vi "Grafici MANAGER.vi"() -> ()   [LabVIEW 2019]
uses:
  TypeDef/Definizione_Grafico_REPORT.ctl
  TypeDef/Definizione_plot.ctl
  Global percorso impostazioni.vi
panel:
  in  "proponi plot":bool
  in  "SALVA plots":bool
  in  "SALVA GRAFICI":bool
  in  "exit":bool
  out "deleted portion":T1[](array[typedef]) {"PLOT"."GRANDEZZA Y" items=["Banco", "Anno", "Numero", "N° tabella", "Misura", "Tipo prova", "Progressivo Acq", "tempo[h:m:s]", "tempo acq[min]", "f [Hz]", "Uav [V]", "Iav [A]", "Tq [Nm]", "n [rpm]", "P1 [kW]", "P1 n[kW]", "Q [m3/h]", "Q n[m3/h]", "Q [l/min]", "Q n[l/min]", "H1 [m]", "Dislivello [m]", "Hdinamica [m]", "HvAsp [m]", "HvMand [m]", "HvTot [m]", "H2 [m]", "Htot [m]", "Htot n[m]", "P3 (Phyd) [kW]", "P3 (Phyd) n[kW]", "P2 [kW]", "P2 n[kW]", "P2 n ps[kW]", "eta motore [%]", "eta pompa [%]", "eta pompa n[%]", "eta gruppo [%]", "eta gruppo n[%]", "T acqua [°C]", "Densità liquido [kg/m3]", "P barometrica [mbar]", "pf", "Uch1 [V]", "Uch2 [V]", "Uch3 [V]", "Ich1 [A]", "Ich2 [A]", "Ich3 [A]", "Temp.amb[°C]", "Ru-w [ohm]", "DTavvolg. [°C]", "Tamb Freddo [°C]", "Ru-w Freddo [ohm]", "Tc1[°C]", "Tc2[°C]", "Tc3[°C]", "Tc4[°C]", "Tc5", "Tc6", "Tc7", "Tc8", "H1[Bar]", "H2[bar]", "P premist.[Bar]", "Pserb[bar]", "n°NPSH", "NPSH", "Htot Ref[m]", "NPSH_%caduta", "%caduta", "Qref [m3/h]", "MEI"]; "PLOT"."GRANDEZZA X" items=["Banco", "Anno", "Numero", "N° tabella", "Misura", "Tipo prova", "Progressivo Acq", "tempo[h:m:s]", "tempo acq[min]", "f [Hz]", "Uav [V]", "Iav [A]", "Tq [Nm]", "n [rpm]", "P1 [kW]", "P1 n[kW]", "Q [m3/h]", "Q n[m3/h]", "Q [l/min]", "Q n[l/min]", "H1 [m]", "Dislivello [m]", "Hdinamica [m]", "HvAsp [m]", "HvMand [m]", "HvTot [m]", "H2 [m]", "Htot [m]", "Htot n[m]", "P3 (Phyd) [kW]", "P3 (Phyd) n[kW]", "P2 [kW]", "P2 n[kW]", "P2 n ps[kW]", "eta motore [%]", "eta pompa [%]", "eta pompa n[%]", "eta gruppo [%]", "eta gruppo n[%]", "T acqua [°C]", "Densità liquido [kg/m3]", "P barometrica [mbar]", "pf", "Uch1 [V]", "Uch2 [V]", "Uch3 [V]", "Ich1 [A]", "Ich2 [A]", "Ich3 [A]", "Temp.amb[°C]", "Ru-w [ohm]", "DTavvolg. [°C]", "Tamb Freddo [°C]", "Ru-w Freddo [ohm]", "Tc1[°C]", "Tc2[°C]", "Tc3[°C]", "Tc4[°C]", "Tc5", "Tc6", "Tc7", "Tc8", "H1[Bar]", "H2[bar]", "P premist.[Bar]", "Pserb[bar]", "n°NPSH", "NPSH", "Htot Ref[m]", "NPSH_%caduta", "%caduta", "Qref [m3/h]", "MEI"]; "Assi grafico"."ASSE X" items=["X 1", "X 2"]; "Assi grafico"."ASSE Y" items=["Y 1", "Y 2", "Y 3", "Y 4"]}
  out "Array plot":T1[](array[typedef]) {"PLOT"."GRANDEZZA Y" items=["Banco", "Anno", "Numero", "N° tabella", "Misura", "Tipo prova", "Progressivo Acq", "tempo[h:m:s]", "tempo acq[min]", "f [Hz]", "Uav [V]", "Iav [A]", "Tq [Nm]", "n [rpm]", "P1 [kW]", "P1 n[kW]", "Q [m3/h]", "Q n[m3/h]", "Q [l/min]", "Q n[l/min]", "H1 [m]", "Dislivello [m]", "Hdinamica [m]", "HvAsp [m]", "HvMand [m]", "HvTot [m]", "H2 [m]", "Htot [m]", "Htot n[m]", "P3 (Phyd) [kW]", "P3 (Phyd) n[kW]", "P2 [kW]", "P2 n[kW]", "P2 n ps[kW]", "eta motore [%]", "eta pompa [%]", "eta pompa n[%]", "eta gruppo [%]", "eta gruppo n[%]", "T acqua [°C]", "Densità liquido [kg/m3]", "P barometrica [mbar]", "pf", "Uch1 [V]", "Uch2 [V]", "Uch3 [V]", "Ich1 [A]", "Ich2 [A]", "Ich3 [A]", "Temp.amb[°C]", "Ru-w [ohm]", "DTavvolg. [°C]", "Tamb Freddo [°C]", "Ru-w Freddo [ohm]", "Tc1[°C]", "Tc2[°C]", "Tc3[°C]", "Tc4[°C]", "Tc5", "Tc6", "Tc7", "Tc8", "H1[Bar]", "H2[bar]", "P premist.[Bar]", "Pserb[bar]", "n°NPSH", "NPSH", "Htot Ref[m]", "NPSH_%caduta", "%caduta", "Qref [m3/h]", "MEI"]; "PLOT"."GRANDEZZA X" items=["Banco", "Anno", "Numero", "N° tabella", "Misura", "Tipo prova", "Progressivo Acq", "tempo[h:m:s]", "tempo acq[min]", "f [Hz]", "Uav [V]", "Iav [A]", "Tq [Nm]", "n [rpm]", "P1 [kW]", "P1 n[kW]", "Q [m3/h]", "Q n[m3/h]", "Q [l/min]", "Q n[l/min]", "H1 [m]", "Dislivello [m]", "Hdinamica [m]", "HvAsp [m]", "HvMand [m]", "HvTot [m]", "H2 [m]", "Htot [m]", "Htot n[m]", "P3 (Phyd) [kW]", "P3 (Phyd) n[kW]", "P2 [kW]", "P2 n[kW]", "P2 n ps[kW]", "eta motore [%]", "eta pompa [%]", "eta pompa n[%]", "eta gruppo [%]", "eta gruppo n[%]", "T acqua [°C]", "Densità liquido [kg/m3]", "P barometrica [mbar]", "pf", "Uch1 [V]", "Uch2 [V]", "Uch3 [V]", "Ich1 [A]", "Ich2 [A]", "Ich3 [A]", "Temp.amb[°C]", "Ru-w [ohm]", "DTavvolg. [°C]", "Tamb Freddo [°C]", "Ru-w Freddo [ohm]", "Tc1[°C]", "Tc2[°C]", "Tc3[°C]", "Tc4[°C]", "Tc5", "Tc6", "Tc7", "Tc8", "H1[Bar]", "H2[bar]", "P premist.[Bar]", "Pserb[bar]", "n°NPSH", "NPSH", "Htot Ref[m]", "NPSH_%caduta", "%caduta", "Qref [m3/h]", "MEI"]; "Assi grafico"."ASSE X" items=["X 1", "X 2"]; "Assi grafico"."ASSE Y" items=["Y 1", "Y 2", "Y 3", "Y 4"]}
  out "Array grafici":T2[](array[typedef]) {"ASSE Y 5"."Decimali" min=0 max=6; "ASSE Y 4"."Decimali" min=0 max=6; "ASSE Y 3"."Decimali" min=0 max=6; "ASSE Y 2"."Decimali" min=0 max=6; "ASSE Y 1"."Decimali" min=0 max=6; "ASSE X 2"."Decimali" min=0 max=6; "ASSE X 1"."Decimali" min=0 max=6}
  in  "Tab Control":enum32{"GESTIONE GRAFICI"}(tab)
  in  "carica plot":bool
  in  "CARICA PLOT GRAFICI":bool
  in  "ELIMINA PLOT":bool
  in  "ELIMINA GRAFICO":bool
  in  "carica grafico":bool
  in  "lista grafici":i32(listbox) caption="LISTA GRAFICI ESISTENTI"
  in  "CREA GRAFICO":bool
  in  "GRAFICO":T2 {"ASSE Y 5"."Decimali" min=0 max=6; "ASSE Y 4"."Decimali" min=0 max=6; "ASSE Y 3"."Decimali" min=0 max=6; "ASSE Y 2"."Decimali" min=0 max=6; "ASSE Y 1"."Decimali" min=0 max=6; "ASSE X 2"."Decimali" min=0 max=6; "ASSE X 1"."Decimali" min=0 max=6}
  in  "PLOT":T1={"Assi grafico"={"ASSE Y"=0, "ASSE X"=0, "Colore x"=0, "Colore y"=0}, "TIPO COLLEGAMENTO"="", "PLOT"={"GRANDEZZA X"=0, "GRANDEZZA Y"=16, "COLORE PLOT"=0, "NOME PLOT"="", "Larghezza linea"=0, "stile linea"=0, "stile punto"=0}, "NOME GRAFICO"=""} {"PLOT"."GRANDEZZA Y" items=["Banco", "Anno", "Numero", "Ntabella", "Misura", "Tipo Prova", "ProgressivoAcq", "Descrizione", "Data_ora", "t. acq [h:m:s]", "t. acq [min]", "t. acq [s]", "n [rpm]", "f [Hz]", "U1[V]", "U2 [V]", "U3 [V]", "U123_media [V]", "I1[A]", "I2[A]", "I3[A]", "I123_media [A]*I", "I_123_sbil [%]", "pf", "P1 [W]", "P1 [kW]", "Q [VAR]", "Q [kVAR]", "S [VA]", "S [kVA]", "C [Nm]*C", "Cric [Nm]", "Cric\\Cnom", "Iric[A]", "Iric\\Inom", "P2_mecc [W]", "P2_mecc [kW]", "eta motore [%]", "Scorr[%]", "Tamb[°C]", "R1[ohm]", "R2[ohm]", "R3[ohm]", "DT_R1[°C]", "DT_R2[°C]", "DT_R3[°C]", "TambFreddo[°C]", "R1_freddo[ohm]", "R2_freddo[ohm]", "R3_freddo[ohm]", "DEO[mm\\s]", "DEO[ge]", "DEV[mm\\s]", "DEV[ge]", "NDEO[mm\\s]", "NDEO[ge]", "NDEV[mm\\s]", "NDEV[ge]", "ASS.[mm\\s]", "ASS.[ge]", "TC1[°C]", "TC2[°C]", "TC3[°C]"]; "PLOT"."GRANDEZZA X" items=["Banco", "Anno", "Numero", "Ntabella", "Misura", "Tipo Prova", "ProgressivoAcq", "Descrizione", "Data_ora", "t. acq [h:m:s]", "t. acq [min]", "t. acq [s]", "n [rpm]", "f [Hz]", "U1[V]", "U2 [V]", "U3 [V]", "U123_media [V]", "I1[A]", "I2[A]", "I3[A]", "I123_media [A]*I", "I_123_sbil [%]", "pf", "P1 [W]", "P1 [kW]", "Q [VAR]", "Q [kVAR]", "S [VA]", "S [kVA]", "C [Nm]*C", "Cric [Nm]", "Cric\\Cnom", "Iric[A]", "Iric\\Inom", "P2_mecc [W]", "P2_mecc [kW]", "eta motore [%]", "Scorr[%]", "Tamb[°C]", "R1[ohm]", "R2[ohm]", "R3[ohm]", "DT_R1[°C]", "DT_R2[°C]", "DT_R3[°C]", "TambFreddo[°C]", "R1_freddo[ohm]", "R2_freddo[ohm]", "R3_freddo[ohm]", "DEO[mm\\s]", "DEO[ge]", "DEV[mm\\s]", "DEV[ge]", "NDEO[mm\\s]", "NDEO[ge]", "NDEV[mm\\s]", "NDEV[ge]", "ASS.[mm\\s]", "ASS.[ge]", "TC1[°C]", "TC2[°C]", "TC3[°C]"]; "Assi grafico"."ASSE X" items=["RPM"]; "Assi grafico"."ASSE Y" items=["C[Nm]"]}
  in  "lista plot":i32(listbox) caption="LISTA PLOT"
  in  "Add plot":bool
  in  "Y Scale.Visible":bool
  in  "Active Y Scale":i32
  in  "X Scale.Visible":bool
  in  "Active X Scale":i32
  out "CURVE IDRAULICHE QH":cluster{"X":dbl[], "Y":dbl[]}[](graph)
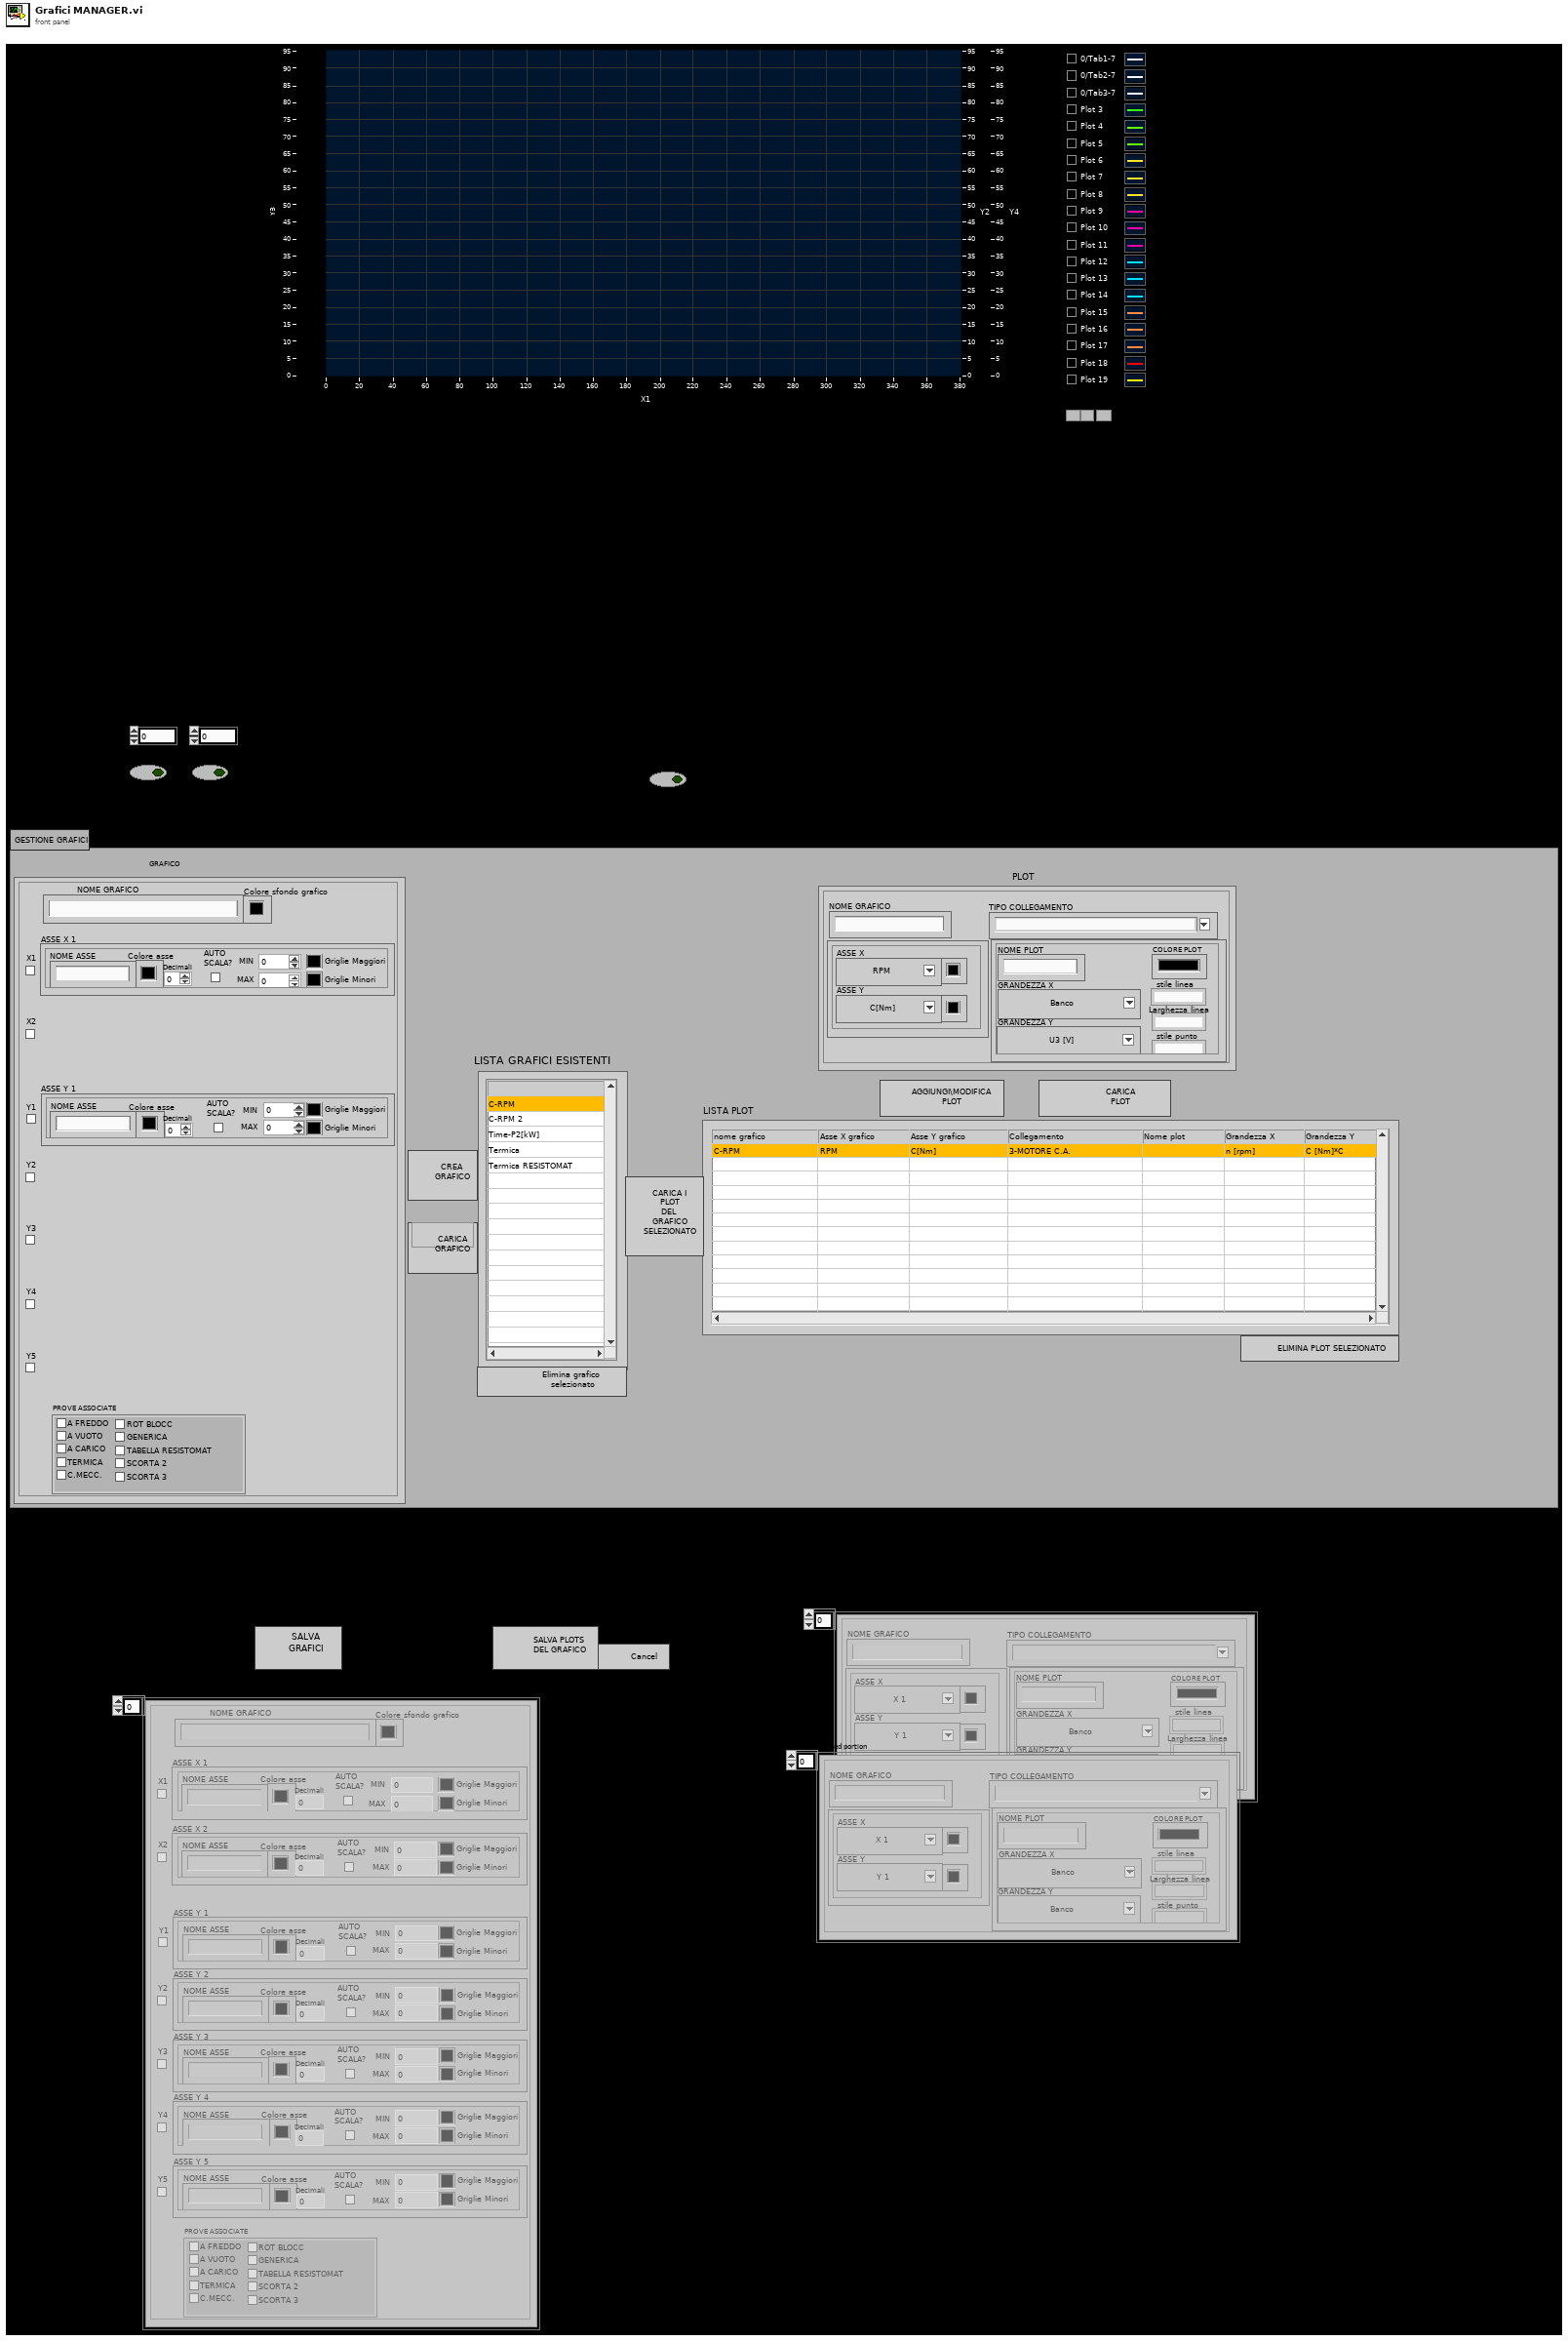
[diagram p1: front panel]
types:
  T1 = typedef "Definizione_plot.ctl" = cluster{"Assi grafico":cluster{"ASSE Y":u16, "ASSE X":u16, "Colore x":u32, "Colore y":u32}, "TIPO COLLEGAMENTO":string, "PLOT":cluster{"GRANDEZZA X":u16, "GRANDEZZA Y":u16, "COLORE PLOT":u32, "NOME PLOT":string, "Larghezza linea":u16, "stile linea":u16, "stile punto":u16}, "NOME GRAFICO":string}
  T2 = typedef "Definizione_Grafico_REPORT.ctl" = cluster{"ASSE X 1":cluster{"NOME ASSE":string, "AUTO\nSCALA?":bool, "MIN":dbl, "MAX":dbl, "Colore asse":u32, "Griglie Maggiori":u32, "Griglie Minori":u32, "Decimali":i8}, "ASSE X 2":cluster{"NOME ASSE":string, "AUTO\nSCALA?":bool, "MIN":dbl, "MAX":dbl, "Colore asse":u32, "Griglie Maggiori":u32, "Griglie Minori":u32, "Decimali":i8}, "ASSE Y 1":cluster{"NOME ASSE":string, "AUTO\nSCALA?":bool, "MIN":dbl, "MAX":dbl, "Colore asse":u32, "Griglie Maggiori":u32, "Griglie Minori":u32, "Decimali":i8}, "ASSE Y 2":cluster{"NOME ASSE":string, "AUTO\nSCALA?":bool, "MIN":dbl, "MAX":dbl, "Colore asse":u32, "Griglie Maggiori":u32, "Griglie Minori":u32, "Decimali":i8}, "ASSE Y 3":cluster{"NOME ASSE":string, "AUTO\nSCALA?":bool, "MIN":dbl, "MAX":dbl, "Colore asse":u32, "Griglie Maggiori":u32, "Griglie Minori":u32, "Decimali":i8}, "ASSE Y 4":cluster{"NOME ASSE":string, "AUTO\nSCALA?":bool, "MIN":dbl, "MAX":dbl, "Colore asse":u32, "Griglie Maggiori":u32, "Griglie Minori":u32, "Decimali":i8}, "X1":bool, "X2":bool, "Y1":bool, "Y2":bool, "Y3":bool, "Y4":bool, "NOME GRAFICO":string, "PROVE ASSOCIATE":cluster{"A FREDDO":bool, "A VUOTO":bool, "A CARICO":bool, "TERMICA":bool, "C.MECC.":bool, "ROT BLOCC":bool, "GENERICA":bool, "TABELLA RESISTOMAT":bool, "SCORTA 2":bool, "SCORTA 3":bool}, "ASSE Y 5":cluster{"NOME ASSE":string, "AUTO\nSCALA?":bool, "MIN":dbl, "MAX":dbl, "Colore asse":u32, "Griglie Maggiori":u32, "Griglie Minori":u32, "Decimali":i8}, "Y5":bool, "Colore sfondo grafico":u32}
  T3 = enum16{"open", "replace", "create", "open or create", "replace or create", "replace or create with confirmation"}
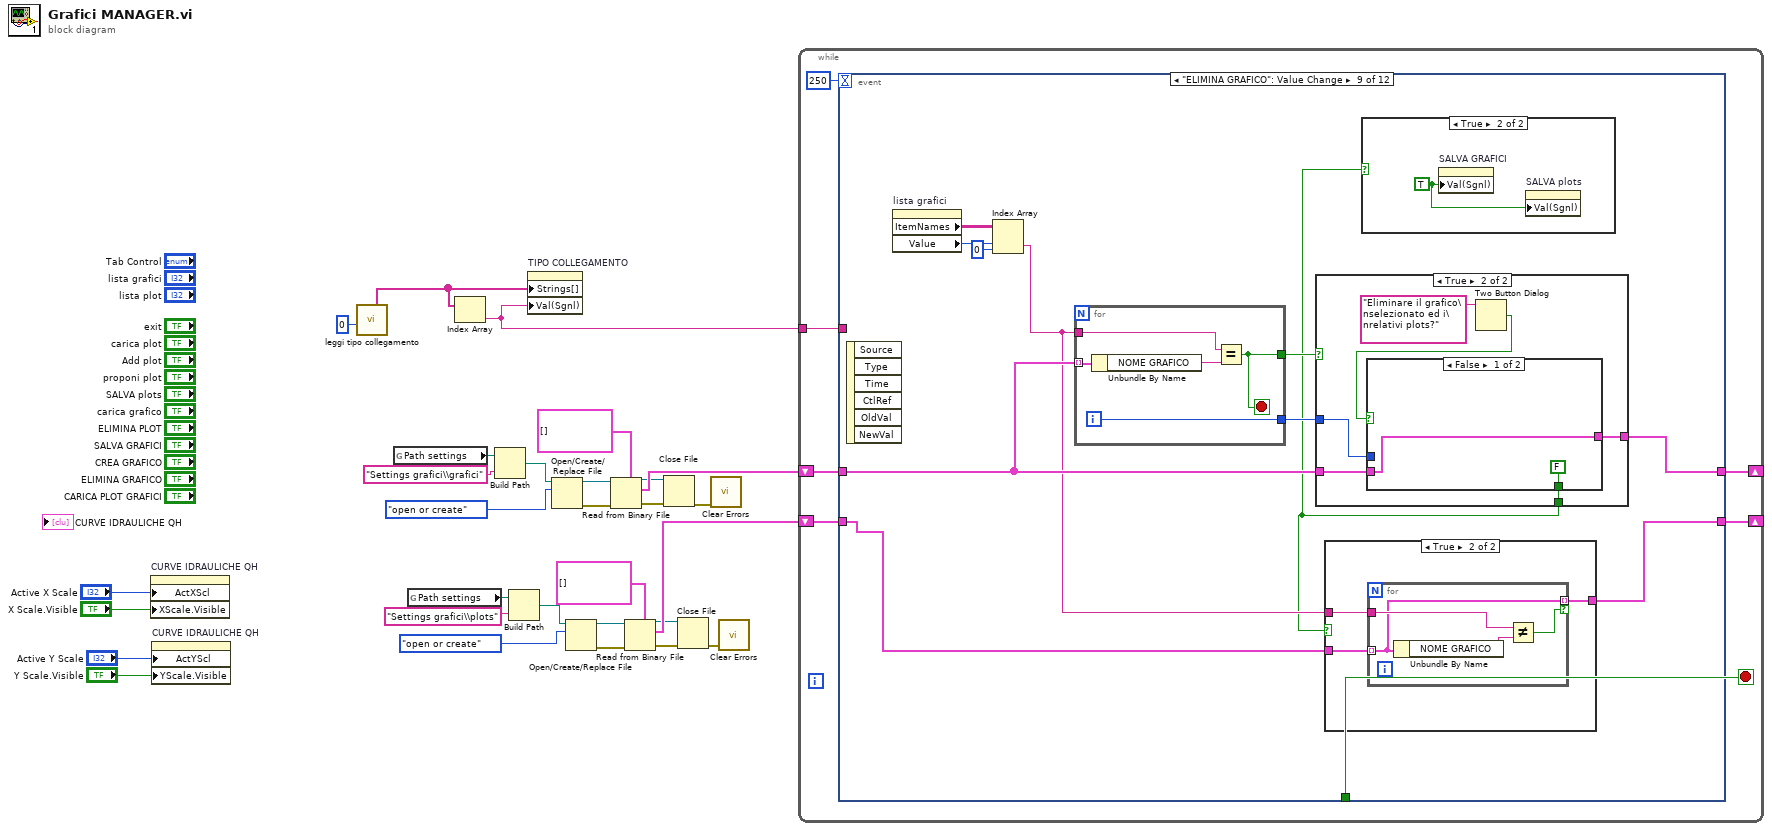
[diagram p0: block diagram]
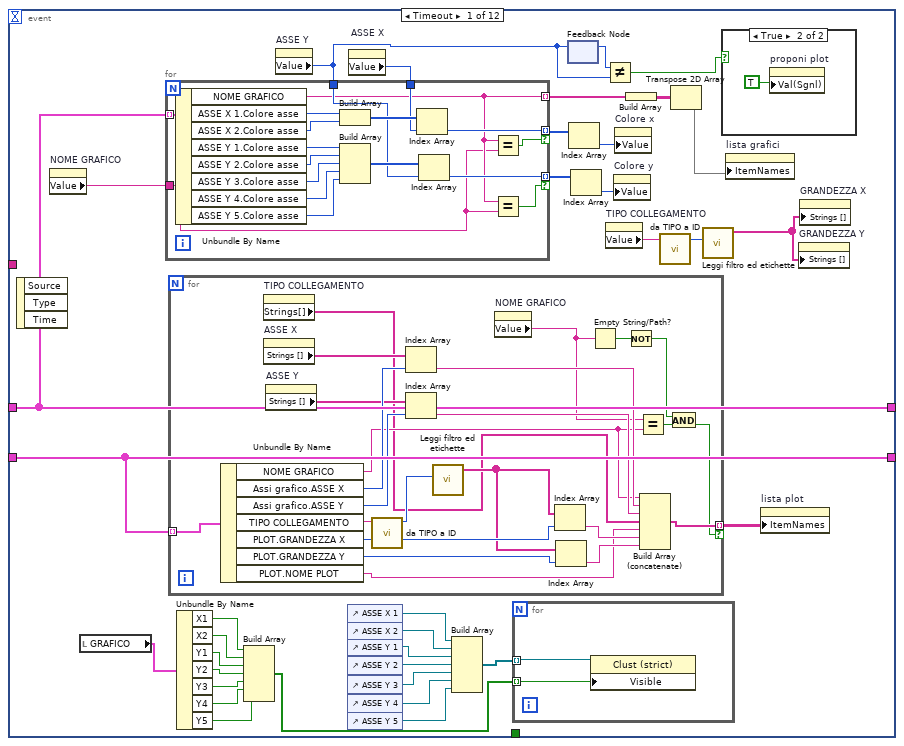
[diagram p2: hidden frame]
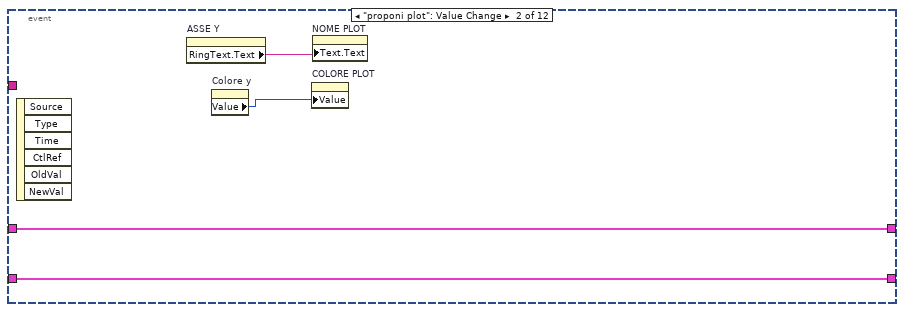
[diagram p4: hidden frame]
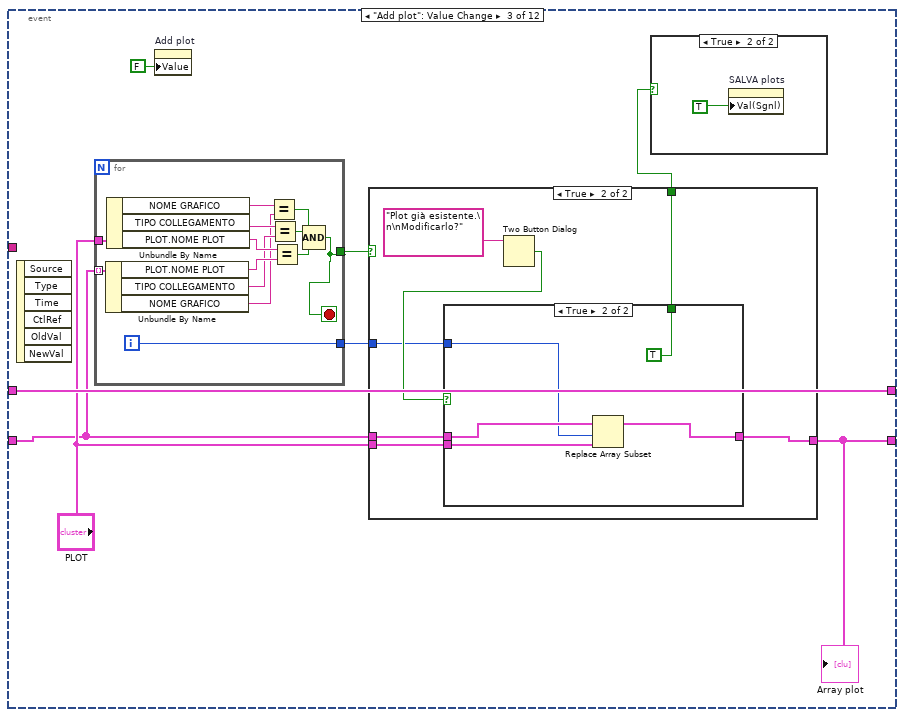
[diagram p5: hidden frame]
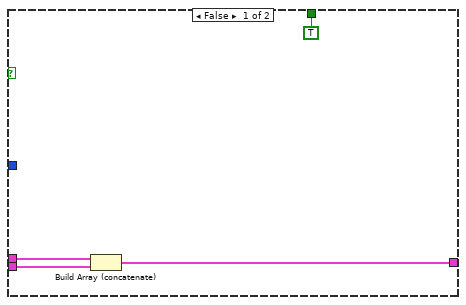
[diagram p7: hidden frame]
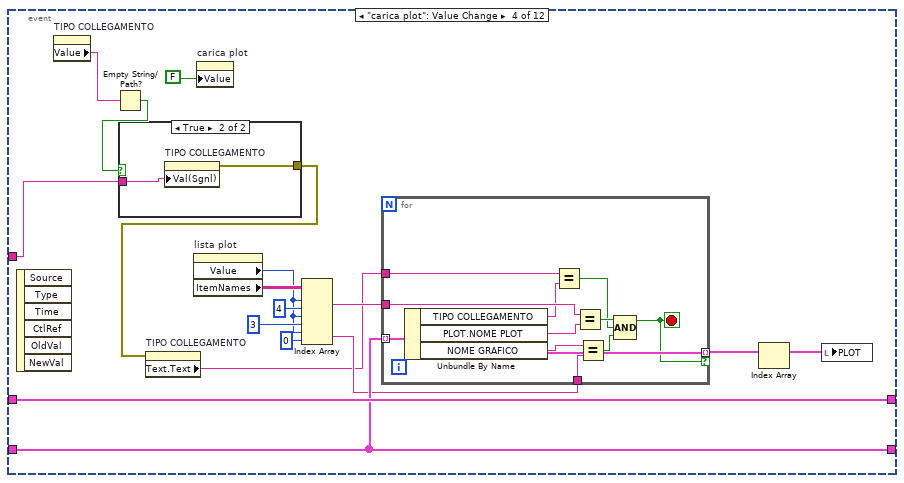
[diagram p9: hidden frame]
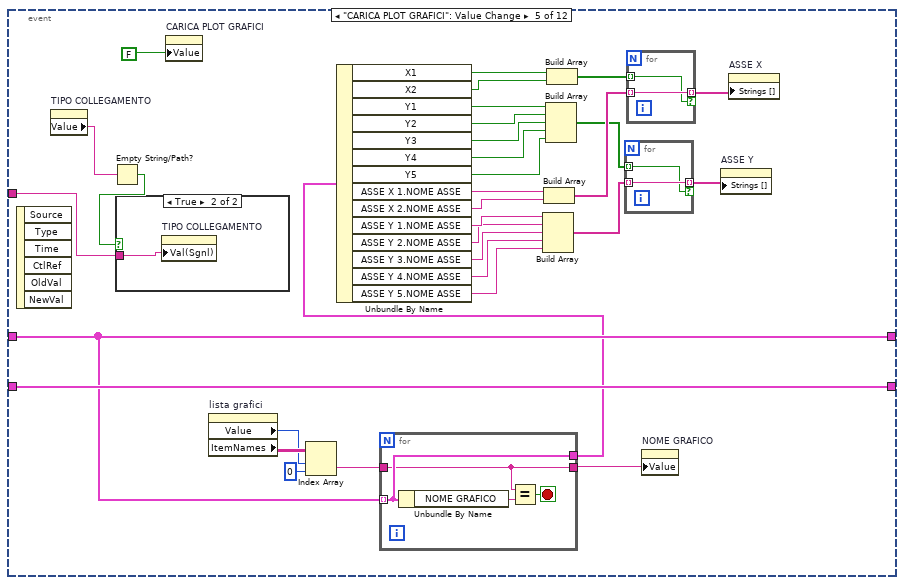
[diagram p11: hidden frame]
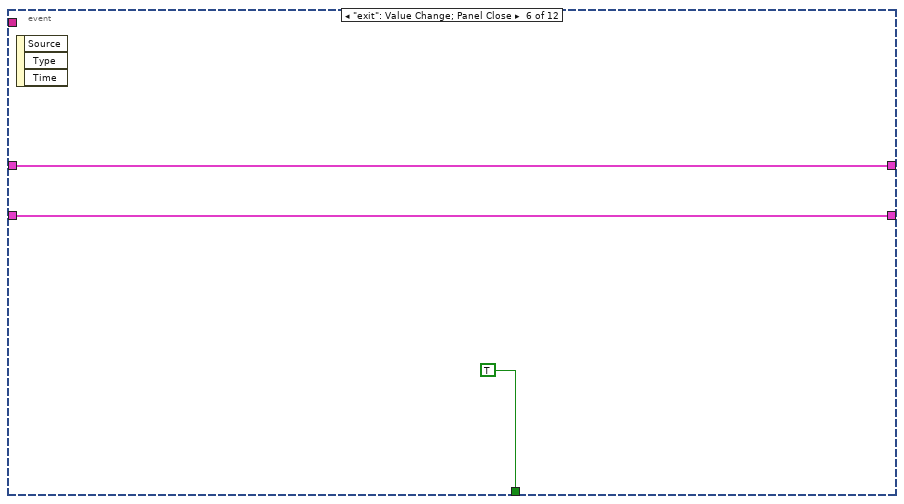
[diagram p13: hidden frame]
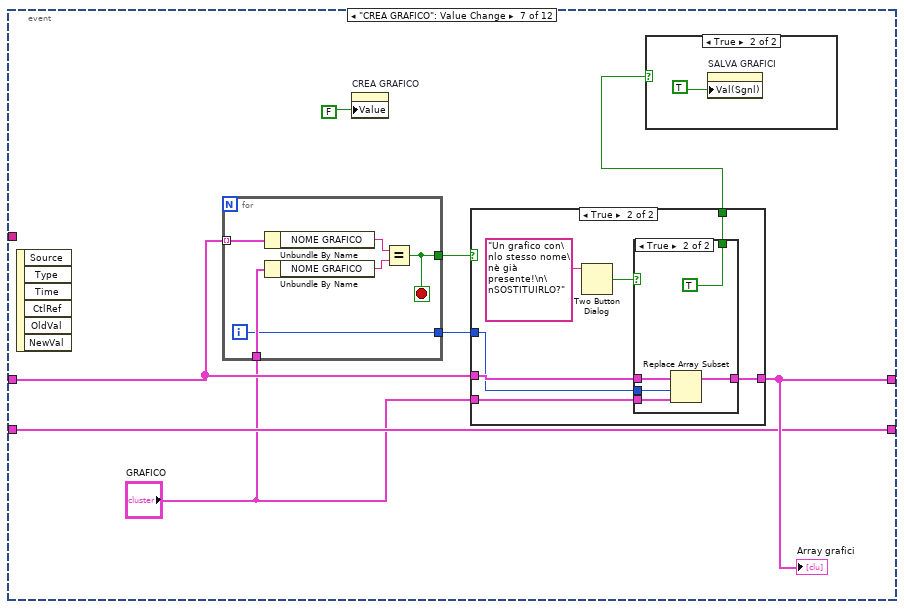
[diagram p14: hidden frame]
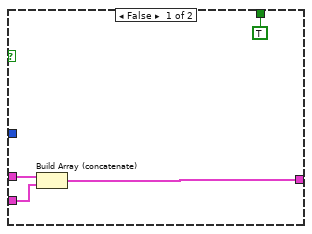
[diagram p16: hidden frame]
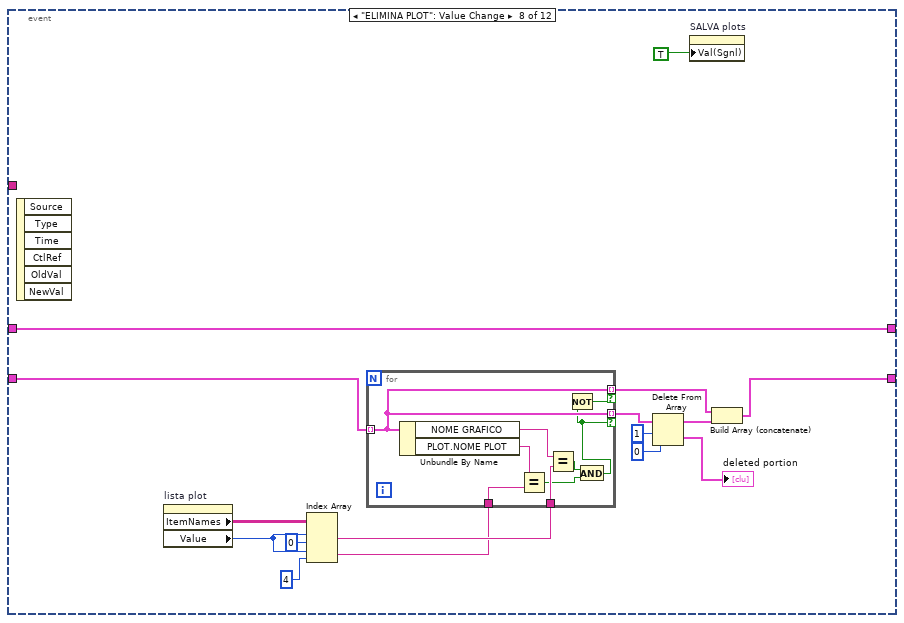
[diagram p18: hidden frame]
diagram:
  n1 = property on="CURVE IDRAULICHE QH" class="XYGraph (strict)"("ActXScl"="Active X Scale", "XScale.Visible"="X Scale.Visible") -> ()  [unwired: 2 in, 2 out]
  n2 = property on="CURVE IDRAULICHE QH" class="XYGraph (strict)"("ActYScl"="Active Y Scale", "YScale.Visible"="Y Scale.Visible") -> ()  [unwired: 2 in, 2 out]
  n3 = call "leggi tipo collegamento.vi"("lingua"=0) -> ("lista"=w2:string[])  [unwired: 5 in, 5 out]
  n4 = global read "Global percorso impostazioni.vi" "Path settings"() -> (w19:path)
  n5 = global read "Global percorso impostazioni.vi" "Path settings"() -> (w9:path)
  n6 = Index Array(array=w2) -> (element=w1:string)  [unwired: 1 in]
  n7 = Build Path(base path=w19, name or relative path="Settings grafici\\grafici") -> (appended path=w18:path)
  n8 = Build Path(base path=w9, name or relative path="Settings grafici\\plots") -> (appended path=w10:path)
  n9 = property on="TIPO COLLEGAMENTO" class="CmbBox"("Strings[]"=w2, "Val(Sgnl)"=w1) -> ()  [unwired: 2 in, 2 out]
  n10 = Open/Create/Replace File(file path (use dialog)=w18, operation (0:open)=T3."open or create") -> (refnum out=w16:refnum<file>, error out=w15:errorcluster)  [unwired: 4 in, 1 out]
  n11 = Open/Create/Replace File(file path (use dialog)=w10, operation (0:open)=T3."open or create") -> (refnum out=w12:refnum<file>, error out=w13:errorcluster)  [unwired: 4 in, 1 out]
  n12 = Read from Binary File(5:T2[] [], 8:w15, 11:w16) -> (0:w21:errorcluster, 2:w24:T2[], 3:w22:refnum<file>)  [unwired: 3 in, 1 out]
  n13 = Read from Binary File(5:T1[] [], 8:w13, 11:w12) -> (0:w7:errorcluster, 2:w23:T1[], 3:w6:refnum<file>)  [unwired: 3 in, 1 out]
  n14 = Close File(refnum=w22, error in=w21) -> (error out=w4:errorcluster)  [unwired: 1 out]
  n15 = Close File(refnum=w6, error in=w7) -> (error out=w3:errorcluster)  [unwired: 1 out]
  n16 = call <vilib>:"Clear Errors.vi"("error in (no error)"=w4) -> ()  [unwired: 5 in, 2 out]
  n17 = call <vilib>:"Clear Errors.vi"("error in (no error)"=w3) -> ()  [unwired: 5 in, 2 out]
  n18 = while {
    shift-right: [w35] -> _
    shift-left: w24 -> [w36]
    shift-right: [w32] -> _
    shift-left: w23 -> [w31]
    tunnel: w1 -> [w30]
    stop <- w34 stop-if-true
    n19 = event shown="[8] \"ELIMINA GRAFICO\": Value Change" {
      selector: _ -> [_ _ _ _ _ _ _ _ _ _ _ _]
      dyn-events: _ -> [_ _ _ _ _ _ _ _ _ _ _ _]
      timeout: 250 -> [_ _ _ _ _ _ _ _ _ _ _ _]
      tunnel: w36 -> [w71 w119 w126 w175 w215 w231 w238 w280 w296 w332 w343 w360]
      tunnel: [w71 w119 w126 w175 w215 w231 w240 w280 w295 w332 w343 w360] -> w35
      tunnel: [_ _ _ _ _ TRUE _ _ _ _ _ _] -> w34
      tunnel: [w66 w118 w127 w172 w217 w230 w239 w272 w291 w336 w350 w351] -> w32
      tunnel: w31 -> [w66 w118 w124 w172 w217 w230 w239 w277 w292 w336 w350 w351]
      tunnel: w30 -> [_ _ _ w160 w189 _ _ _ _ _ _ _]
      event Timeout {
        n20 = event-data() -> ()  [unwired: 1 in, 3 out]
        n21 = property on="NOME GRAFICO" class="Str"() -> ("Value"=w47:string)  [unwired: 2 in, 2 out]
        n22 = local read "GRAFICO"() -> (w64:T2)
        n23 = for {
          tunnel: w66 -> [w97] mode=indexing
          tunnel: [w94] -> w65 mode=indexing if=w76
          n24 = Unbundle By Name(w97) -> ("NOME GRAFICO"=w84:string, "Assi grafico.ASSE X"=w92:u16, "Assi grafico.ASSE Y"=w89:u16, "TIPO COLLEGAMENTO"=w81:string, "PLOT.GRANDEZZA X"=w96:u16, "PLOT.GRANDEZZA Y"=w95:u16, "PLOT.NOME PLOT"=w85:string)
          n25 = property on="TIPO COLLEGAMENTO" class="CmbBox"() -> ("Strings[]"=w79:string[])  [unwired: 2 in, 2 out]
          n26 = property on="ASSE X" class="Ring (strict)"() -> ("Strings []"=w93:string[])  [unwired: 2 in, 2 out]
          n27 = property on="ASSE Y" class="Ring (strict)"() -> ("Strings []"=w90:string[])  [unwired: 2 in, 2 out]
          n28 = call "da TIPO a ID.vi"("TIPO"=w81) -> ("ID"=w80:i32)  [unwired: 10 in]
          n29 = Index Array(array=w93, index=w92) -> (element=w91:string)
          n30 = Index Array(array=w90, index=w89) -> (element=w88:string)
          n31 = call "Leggi filtro ed etichette.vi"("ID COLLEGAMENTO"=w80) -> ("ETICHETTE"=w82:string[])  [unwired: 5 in, 5 out]
          n32 = property on="NOME GRAFICO" class="Str"() -> ("Value"=w78:string)  [unwired: 2 in, 2 out]
          n33 = Index Array(array=w82, index=w96) -> (element=w86:string)
          n34 = Index Array(array=w82, index=w95) -> (element=w87:string)
          n35 = Empty String/Path?(string/path=w78) -> (empty?=w77:bool)
          n36 = Not(x=w77) -> (.not. x?=w75:bool)
          n37 = Equal?(x=w78, y=w84) -> (x = y?=w83:bool)
          n38 = Build Array (concatenate)(w84, w91, w88, w79, w85, w86, w87) -> (w94:string[])
          n39 = And(x=w75, y=w83) -> (x .and. y?=w76:bool)
        }
        n40 = Unbundle By Name(w64) -> ("X1"=w63:bool, "X2"=w62:bool, "Y1"=w61:bool, "Y2"=w60:bool, "Y3"=w59:bool, "Y4"=w58:bool, "Y5"=w49:bool)
        n41 = Build Array(w63, w62, w61, w60, w59, w58, w49) -> (w50:bool[])
        n42 = property on="ASSE Y" class="Ring (strict)"() -> ("Value"=w40:u16)  [unwired: 2 in, 2 out]
        n43 = control-ref of="ASSE X 1"() -> (w57:refnum<vi>)
        n44 = control-ref of="ASSE X 2"() -> (w56:refnum<vi>)
        n45 = control-ref of="ASSE Y 1"() -> (w55:refnum<vi>)
        n46 = control-ref of="ASSE Y 2"() -> (w54:refnum<vi>)
        n47 = control-ref of="ASSE Y 3"() -> (w53:refnum<vi>)
        n48 = control-ref of="ASSE Y 4"() -> (w52:refnum<vi>)
        n49 = control-ref of="ASSE Y 5"() -> (w48:refnum<vi>)
        n50 = property on="ASSE X" class="Ring (strict)"() -> ("Value"=w46:u16)  [unwired: 2 in, 2 out]
        n51 = for {
          tunnel: w71 -> [w115] mode=indexing
          tunnel: [w99] -> w70 mode=indexing
          tunnel: w47 -> [w98]
          tunnel: w46 -> [w105]
          tunnel: w40 -> [w104]
          tunnel: [w103] -> w45 mode=indexing if=w100
          tunnel: [w102] -> w44 mode=indexing if=w101
          n52 = Unbundle By Name(w115) -> ("NOME GRAFICO"=w99:string, "ASSE X 1.Colore asse"=w114:u32, "ASSE X 2.Colore asse"=w113:u32, "ASSE Y 1.Colore asse"=w112:u32, "ASSE Y 2.Colore asse"=w111:u32, "ASSE Y 3.Colore asse"=w110:u32, "ASSE Y 4.Colore asse"=w109:u32, "ASSE Y 5.Colore asse"=w108:u32)
          n53 = Build Array(w114, w113) -> (w107:u32[])
          n54 = Build Array(w112, w111, w110, w109, w108) -> (w106:u32[])
          n55 = Index Array(array=w107, index=w105) -> (element=w103:u32)
          n56 = Index Array(array=w106, index=w104) -> (element=w102:u32)
          n57 = Equal?(x=w99, y=w98) -> (x = y?=w100:bool)
          n58 = Equal?(x=w99, y=w98) -> (x = y?=w101:bool)
        }
        n59 = Build Array(w57, w56, w55, w54, w53, w52, w48) -> (w51:refnum<vi>[])
        n60 = for {
          tunnel: w51 -> [w74] mode=indexing
          tunnel: w50 -> [w73] mode=indexing
          n61 = property class="Clust (strict)"(reference=w74, "Visible"=w73) -> ()  [unwired: 1 in, 2 out]
        }
        n62 = feedback-in #1(w40) -> ()
        n63 = feedback #1() -> (w41:u16)  [unwired: 1 in]
        n64 = Index Array(array=w45) -> (element=w43:u32)  [unwired: 1 in]
        n65 = Index Array(array=w44) -> (element=w42:u32)  [unwired: 1 in]
        n66 = Not Equal?(x=w41, y=w40) -> (x != y?=w39:bool)
        n67 = property on="TIPO COLLEGAMENTO" class="CmbBox"() -> ("Value"=w38:string)  [unwired: 2 in, 2 out]
        n68 = property on="Colore y" class="ColBox"("Value"=w42) -> ()  [unwired: 2 in, 2 out]
        n69 = property on="Colore x" class="ColBox"("Value"=w43) -> ()  [unwired: 2 in, 2 out]
        n70 = Build Array(w70) -> (w69:string[][])
        n71 = call "da TIPO a ID.vi"("TIPO"=w38) -> ("ID"=w37:i32)  [unwired: 10 in]
        n72 = Transpose 2D Array(2D array=w69) -> (transposed array=w68:string[][])
        n73 = call "Leggi filtro ed etichette.vi"("ID COLLEGAMENTO"=w37) -> ("ETICHETTE"=w67:string[])  [unwired: 5 in, 5 out]
        n74 = case shown="True" w39 {
          frame False {
          }
          frame True {
            n75 = property on="proponi plot" class="Bool (strict)"("Val(Sgnl)"=TRUE) -> ()  [unwired: 2 in, 2 out]
          }
        }
        n76 = property on="lista grafici" class="MCListbox (strict)"("ItemNames"=w68) -> ()  [unwired: 2 in, 2 out]
        n77 = property on="lista plot" class="MCListbox (strict)"("ItemNames"=w65) -> ()  [unwired: 2 in, 2 out]
        n78 = property on="GRANDEZZA Y" class="Ring (strict)"("Strings []"=w67) -> ()  [unwired: 2 in, 2 out]
        n79 = property on="GRANDEZZA X" class="Ring (strict)"("Strings []"=w67) -> ()  [unwired: 2 in, 2 out]
      }
      event "proponi plot": Value Change {
        n80 = event-data() -> ()  [unwired: 1 in, 6 out]
        n81 = property on="ASSE Y" class="Ring (strict)"() -> ("RingText.Text"=w117:string)  [unwired: 2 in, 2 out]
        n82 = property on="Colore y" class="ColBox"() -> ("Value"=w116:u32)  [unwired: 2 in, 2 out]
        n83 = property on="COLORE PLOT" class="ColBox"("Value"=w116) -> ()  [unwired: 2 in, 2 out]
        n84 = property on="NOME PLOT" class="Str"("Text.Text"=w117) -> ()  [unwired: 2 in, 2 out]
      }
      event "Add plot": Value Change {
        n85 = event-data() -> ()  [unwired: 1 in, 6 out]
        n86 = for {
          tunnel: "PLOT" -> [w157]
          tunnel: w124 -> [w158] mode=indexing
          tunnel: [w149] -> w123
          tunnel: [w154] -> w122
          i -> [w154]
          stop <- w149 stop-if-true
          n87 = Unbundle By Name(w158) -> ("PLOT.NOME PLOT"=w156:string, "TIPO COLLEGAMENTO"=w152:string, "NOME GRAFICO"=w147:string)
          n88 = Unbundle By Name(w157) -> ("NOME GRAFICO"=w148:string, "TIPO COLLEGAMENTO"=w153:string, "PLOT.NOME PLOT"=w155:string)
          n89 = Equal?(x=w148, y=w147) -> (x = y?=w146:bool)
          n90 = Equal?(x=w153, y=w152) -> (x = y?=w150:bool)
          n91 = Equal?(x=w155, y=w156) -> (x = y?=w151:bool)
          n92 = Compound Arithmetic op=AND(w146, w150, w151) -> (w149:bool)
        }
        n93 = property on="Add plot" class="Bool (strict)"("Value"=FALSE ("Add plot")) -> ()  [unwired: 2 in, 2 out]
        n94 = case shown="True" w123 {
          tunnel: [w132 w136] -> w127
          tunnel: "PLOT" -> [w131 w134]
          tunnel: w124 -> [w130 w137]
          tunnel: w122 -> [_ w135]
          tunnel: [TRUE w133] -> w121
          frame False {
            n95 = Build Array (concatenate)(w130, w131) -> (w132:T1[])
          }
          frame True {
            n96 = Two Button Dialog(message="Plot già esistente.\n\nModificarlo?") -> (T button?=w138:bool)  [unwired: 2 in]
            n97 = case shown="True" w138 {
              tunnel: w137 -> [w140 w145]
              tunnel: [w140 w144] -> w136
              tunnel: w135 -> [_ w143]
              tunnel: w134 -> [_ w142]
              tunnel: [_ TRUE] -> w133
              frame False {
              }
              frame True {
                n98 = Replace Array Subset(array=w145, new element=w142, index=w143) -> (w144:T1[])
              }
            }
          }
        }
        "Array plot" <- w127
        n99 = case shown="True" w121 {
          frame False {
          }
          frame True {
            n100 = property on="SALVA plots" class="Bool (strict)"("Val(Sgnl)"=TRUE) -> ()  [unwired: 2 in, 2 out]
          }
        }
      }
      event "carica plot": Value Change {
        n101 = event-data() -> ()  [unwired: 1 in, 6 out]
        n102 = property on="TIPO COLLEGAMENTO" class="CmbBox"() -> ("Value"=w162:string)  [unwired: 2 in, 2 out]
        n103 = Empty String/Path?(string/path=w162) -> (empty?=w161:bool)
        n104 = case shown="True" w161 {
          tunnel: w160 -> [_ w177]
          tunnel: [_ w176] -> w159
          frame False {
          }
          frame True {
            n105 = property on="TIPO COLLEGAMENTO" class="CmbBox"("Val(Sgnl)"=w177) -> (error out=w176:errorcluster)  [unwired: 2 in, 1 out]
          }
        }
        n106 = property on="TIPO COLLEGAMENTO" class="CmbBox"(error in=w159) -> ("Text.Text"=w164:string)  [unwired: 1 in, 2 out]
        n107 = property on="lista plot" class="MCListbox (strict)"() -> ("Value"=w167:i32, "ItemNames"=w173:string[][])  [unwired: 2 in, 2 out]
        n108 = property on="carica plot" class="Bool (strict)"("Value"=FALSE) -> ()  [unwired: 2 in, 2 out]
        n109 = Index Array(array=w173, index (row) #1=w167, index (col) #1=4 ("disabled index (col)"), index (row) #2=w167, index (col) #2=3 ("disabled index (col)"), index (row) #3=w167, index (col) #3=0 ("disabled index (col)")) -> (element #1=w171:string, element #3=w165:string)  [unwired: 1 out]
        n110 = for {
          tunnel: w172 -> [w186] mode=indexing
          tunnel: w171 -> [w187]
          tunnel: [w186] -> w170 mode=indexing if=w178
          tunnel: w164 -> [w183]
          tunnel: w165 -> [w180]
          stop <- w178 stop-if-true
          n111 = Unbundle By Name(w186) -> ("TIPO COLLEGAMENTO"=w184:string, "PLOT.NOME PLOT"=w188:string, "NOME GRAFICO"=w181:string)
          n112 = Equal?(x=w183, y=w184) -> (x = y?=w182:bool)
          n113 = Equal?(x=w187, y=w188) -> (x = y?=w185:bool)
          n114 = Equal?(x=w181, y=w180) -> (x = y?=w179:bool)
          n115 = Compound Arithmetic op=AND(w185, w182, w179) -> (w178:bool)
        }
        n116 = Index Array(array=w170) -> (element=w163:T1)  [unwired: 1 in]
        n117 = local write "PLOT"(w163) -> ()
      }
      event "CARICA PLOT GRAFICI": Value Change {
        n118 = event-data() -> ()  [unwired: 1 in, 6 out]
        n119 = property on="TIPO COLLEGAMENTO" class="CmbBox"() -> ("Value"=w191:string)  [unwired: 2 in, 2 out]
        n120 = Empty String/Path?(string/path=w191) -> (empty?=w190:bool)
        n121 = case shown="True" w190 {
          tunnel: w189 -> [_ w221]
          frame False {
          }
          frame True {
            n122 = property on="TIPO COLLEGAMENTO" class="CmbBox"("Val(Sgnl)"=w221) -> ()  [unwired: 2 in, 2 out]
          }
        }
        n123 = property on="CARICA PLOT GRAFICI" class="Bool (strict)"("Value"=FALSE) -> ()  [unwired: 2 in, 2 out]
        n124 = property on="lista grafici" class="MCListbox (strict)"() -> ("Value"=w219:i32, "ItemNames"=w220:string[][])  [unwired: 2 in, 2 out]
        n125 = Index Array(array=w220, index (row)=w219, index (col)=0 ("disabled index (col)")) -> (element=w216:string)
        n126 = for {
          tunnel: w215 -> [w227] mode=indexing
          tunnel: w216 -> [w226]
          tunnel: [w227] -> w196
          tunnel: [w226] -> w195
          stop <- w228 stop-if-true
          n127 = Unbundle By Name(w227) -> ("NOME GRAFICO"=w229:string)
          n128 = Equal?(x=w226, y=w229) -> (x = y?=w228:bool)
        }
        n129 = Unbundle By Name(w196) -> ("X1"=w209:bool, "X2"=w208:bool, "Y1"=w213:bool, "Y2"=w212:bool, "Y3"=w211:bool, "Y4"=w210:bool, "Y5"=w193:bool, "ASSE X 1.NOME ASSE"=w206:string, "ASSE X 2.NOME ASSE"=w205:string, "ASSE Y 1.NOME ASSE"=w204:string, "ASSE Y 2.NOME ASSE"=w203:string, "ASSE Y 3.NOME ASSE"=w202:string, "ASSE Y 4.NOME ASSE"=w214:string, "ASSE Y 5.NOME ASSE"=w194:string)
        n130 = Build Array(w204, w203, w202, w214, w194) -> (w198:string[])
        n131 = Build Array(w206, w205) -> (w201:string[])
        n132 = Build Array(w213, w212, w211, w210, w193) -> (w199:bool[])
        n133 = Build Array(w209, w208) -> (w207:bool[])
        n134 = for {
          tunnel: w199 -> [w222] mode=indexing
          tunnel: w198 -> [w223] mode=indexing
          tunnel: [w223] -> w197 mode=indexing if=w222
        }
        n135 = for {
          tunnel: w207 -> [w224] mode=indexing
          tunnel: w201 -> [w225] mode=indexing
          tunnel: [w225] -> w200 mode=indexing if=w224
        }
        n136 = property on="NOME GRAFICO" class="Str"("Value"=w195) -> ()  [unwired: 2 in, 2 out]
        n137 = property on="ASSE Y" class="Ring (strict)"("Strings []"=w197) -> ()  [unwired: 2 in, 2 out]
        n138 = property on="ASSE X" class="Ring (strict)"("Strings []"=w200) -> ()  [unwired: 2 in, 2 out]
      }
      event "exit": Value Change; Panel Close {
        n139 = event-data() -> ()  [unwired: 1 in, 3 out]
      }
      event "CREA GRAFICO": Value Change {
        n140 = event-data() -> ()  [unwired: 1 in, 6 out]
        n141 = for {
          tunnel: w238 -> [w264] mode=indexing
          tunnel: "GRAFICO" -> [w263]
          tunnel: [w260] -> w237
          tunnel: [w259] -> w236
          i -> [w259]
          stop <- w260 stop-if-true
          n142 = Unbundle By Name(w264) -> ("NOME GRAFICO"=w261:string)
          n143 = Unbundle By Name(w263) -> ("NOME GRAFICO"=w262:string)
          n144 = Equal?(x=w261, y=w262) -> (x = y?=w260:bool)
        }
        n145 = property on="CREA GRAFICO" class="Bool (strict)"("Value"=FALSE) -> ()  [unwired: 2 in, 2 out]
        n146 = case shown="True" w237 {
          tunnel: [w245 w249] -> w240
          tunnel: w238 -> [w244 w250]
          tunnel: "GRAFICO" -> [w243 w247]
          tunnel: w236 -> [_ w248]
          tunnel: [TRUE w246] -> w234
          frame False {
            n147 = Build Array (concatenate)(w244, w243) -> (w245:T2[])
          }
          frame True {
            n148 = Two Button Dialog(message="Un grafico con\nlo stesso nome\nè già presente!\n\nSOSTITUIRLO?") -> (T button?=w251:bool)  [unwired: 2 in]
            n149 = case shown="True" w251 {
              tunnel: w250 -> [w253 w258]
              tunnel: [w253 w255] -> w249
              tunnel: w248 -> [_ w257]
              tunnel: w247 -> [_ w256]
              tunnel: [_ TRUE] -> w246
              frame False {
              }
              frame True {
                n150 = Replace Array Subset(array=w258, new element=w256, index=w257) -> (w255:T2[])
              }
            }
          }
        }
        "Array grafici" <- w240
        n151 = case shown="True" w234 {
          frame False {
          }
          frame True {
            n152 = property on="SALVA GRAFICI" class="Bool (strict)"("Val(Sgnl)"=TRUE) -> ()  [unwired: 2 in, 2 out]
          }
        }
      }
      event "ELIMINA PLOT": Value Change {
        n153 = event-data() -> ()  [unwired: 1 in, 6 out]
        n154 = property on="lista plot" class="MCListbox (strict)"() -> ("ItemNames"=w279:string[][], "Value"=w269:i32)  [unwired: 2 in, 2 out]
        n155 = Index Array(array=w279, index (row) #1=w269, index (col) #1=0 ("disabled index (col)"), index (row) #2=w269, index (col) #2=4 ("disabled index (col)")) -> (element #1=w276:string, element #2=w267:string)
        n156 = for {
          tunnel: w277 -> [w288] mode=indexing
          tunnel: w276 -> [w286]
          tunnel: [w288] -> w275 mode=indexing if=w281
          tunnel: [w288] -> w271 mode=indexing if=w287
          tunnel: w267 -> [w284]
          n157 = Unbundle By Name(w288) -> ("NOME GRAFICO"=w289:string, "PLOT.NOME PLOT"=w285:string)
          n158 = Equal?(x=w285, y=w284) -> (x = y?=w282:bool)
          n159 = Equal?(x=w289, y=w286) -> (x = y?=w283:bool)
          n160 = And(x=w283, y=w282) -> (x .and. y?=w281:bool)
          n161 = Not(x=w281) -> (.not. x?=w287:bool)
        }
        n162 = Delete From Array(array=w275, length=1, index=0) -> (deleted portion=→"deleted portion":T1[], array with subset deleted=w273:T1[])
        n163 = property on="SALVA plots" class="Bool (strict)"("Val(Sgnl)"=TRUE) -> ()  [unwired: 2 in, 2 out]
        n164 = Build Array (concatenate)(w271, w273) -> (w272:T1[])
      }
      event "ELIMINA GRAFICO": Value Change {
        n165 = event-data() -> ()  [unwired: 1 in, 6 out]
        n166 = property on="lista grafici" class="MCListbox (strict)"() -> ("ItemNames"=w300:string[][], "Value"=w299:i32)  [unwired: 2 in, 2 out]
        n167 = Index Array(array=w300, index (row)=w299, index (col)=0 ("disabled index (col)")) -> (element=w293:string)
        n168 = for {
          tunnel: w296 -> [w328] mode=indexing
          tunnel: w293 -> [w326]
          tunnel: [w325] -> w294
          tunnel: [w324] -> w297
          i -> [w325]
          stop <- w324 stop-if-true
          n169 = Unbundle By Name(w328) -> ("NOME GRAFICO"=w327:string)
          n170 = Equal?(x=w326, y=w327) -> (x = y?=w324:bool)
        }
        n171 = case shown="True" w297 {
          tunnel: w296 -> [w311 w316]
          tunnel: [w311 w314] -> w295
          tunnel: w294 -> [_ w313]
          tunnel: [FALSE w312] -> w290
          frame False {
          }
          frame True {
            n172 = Two Button Dialog(message="Eliminare il grafico\nselezionato ed i\nrelativi plots?") -> (T button?=w315:bool)  [unwired: 2 in]
            n173 = case shown="False" w315 {
              tunnel: w316 -> [w319 w323]
              tunnel: [w319 w322] -> w314
              tunnel: w313 -> [_ w321]
              tunnel: [FALSE TRUE] -> w312
              frame False {
              }
              frame True {
                n174 = Delete From Array(array=w323, index=w321) -> (array with subset deleted=w322:T2[])  [unwired: 1 in, 1 out]
              }
            }
          }
        }
        n175 = case shown="True" w290 {
          tunnel: w293 -> [_ w305]
          tunnel: w292 -> [w302 w304]
          tunnel: [w302 w303] -> w291
          frame False {
          }
          frame True {
            n176 = for {
              tunnel: w304 -> [w307] mode=indexing
              tunnel: w305 -> [w308]
              tunnel: [w307] -> w303 mode=indexing if=w306
              n177 = Unbundle By Name(w307) -> ("NOME GRAFICO"=w309:string)
              n178 = Not Equal?(x=w308, y=w309) -> (x != y?=w306:bool)
            }
          }
        }
        n179 = case shown="True" w290 {
          frame False {
          }
          frame True {
            w301 = TRUE ("Value (Signaling)")
            n180 = property on="SALVA GRAFICI" class="Bool (strict)"("Val(Sgnl)"=w301) -> ()  [unwired: 2 in, 2 out]
            n181 = property on="SALVA plots" class="Bool (strict)"("Val(Sgnl)"=w301) -> ()  [unwired: 2 in, 2 out]
          }
        }
      }
      event "carica grafico": Value Change {
        n182 = event-data() -> ()  [unwired: 1 in, 6 out]
        n183 = property on="lista grafici" class="MCListbox (strict)"() -> ("Value"=w334:i32, "ItemNames"=w335:string[][])  [unwired: 2 in, 2 out]
        n184 = Index Array(array=w335, index (row)=w334, index (col)=0 ("disabled index (col)")) -> (element=w331:string)
        n185 = for {
          tunnel: w332 -> [w337] mode=indexing
          tunnel: w331 -> [w339]
          tunnel: [w337] -> w330
          stop <- w338 stop-if-true
          n186 = Unbundle By Name(w337) -> ("NOME GRAFICO"=w340:string)
          n187 = Equal?(x=w339, y=w340) -> (x = y?=w338:bool)
        }
        n188 = property on="carica grafico" class="Bool (strict)"("Value"=FALSE) -> ()  [unwired: 2 in, 2 out]
        n189 = local write "GRAFICO"(w330) -> ()
      }
      event "SALVA GRAFICI": Value Change {
        n190 = event-data() -> ()  [unwired: 1 in, 6 out]
        n191 = global read "Global percorso impostazioni.vi" "Path settings"() -> (w345:path)
        n192 = Build Path(base path=w345, name or relative path="Settings grafici\\grafici") -> (appended path=w346:path)
        n193 = Open/Create/Replace File(file path (use dialog)=w346, operation (0:open)=T3."replace or create") -> (refnum out=w348:refnum<file>, error out=w349:errorcluster)  [unwired: 4 in, 1 out]
        n194 = Write to Binary File(file (use dialog)=w348, data=w343, error in=w349) -> (refnum out=w341:refnum<file>, error out=w342:errorcluster)  [unwired: 3 in, 1 out]
        n195 = Close File(refnum=w341, error in=w342) -> ()  [unwired: 2 out]
      }
      event "SALVA plots": Value Change {
        n196 = event-data() -> ()  [unwired: 1 in, 6 out]
        n197 = global read "Global percorso impostazioni.vi" "Path settings"() -> (w355:path)
        n198 = Build Path(base path=w355, name or relative path="Settings grafici\\plots") -> (appended path=w356:path)
        n199 = Open/Create/Replace File(file path (use dialog)=w356, operation (0:open)=T3."replace or create") -> (refnum out=w358:refnum<file>, error out=w359:errorcluster)  [unwired: 4 in, 1 out]
        n200 = Write to Binary File(file (use dialog)=w358, data=w351, error in=w359) -> (refnum out=w352:refnum<file>, error out=w353:errorcluster)  [unwired: 3 in, 1 out]
        n201 = Close File(refnum=w352, error in=w353) -> ()  [unwired: 2 out]
      }
    }
  }
